vi "Read.ProcessData.vi"(8 "error in (no error)":errorcluster, 10 "timeout ms":i32=100, 11 "Read in":refnum<class "Read.lvclass">) -> (0 "error out":errorcluster, 1 "Timeout?":bool, 2 "Data":dbl[](array[numeric]), 3 "Read out":refnum<class "Read.lvclass">)   [LabVIEW 2015, in "Data Access API.lvlib" / "Read.lvclass"]
uses:
  Read.lvclass
  Read.lvclass/Read.ctl
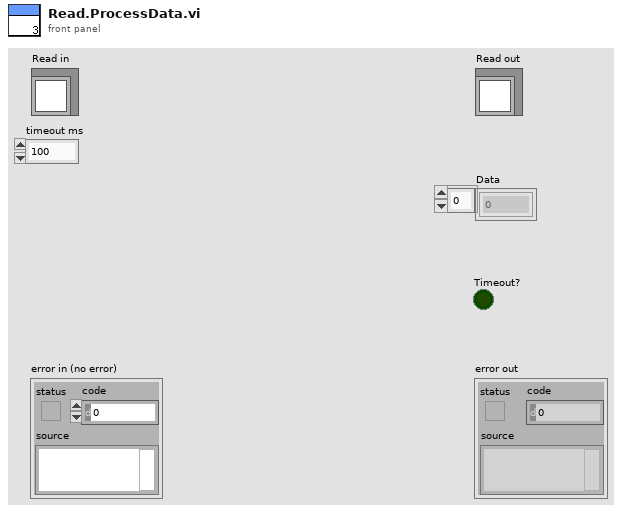
[diagram p1: front panel]
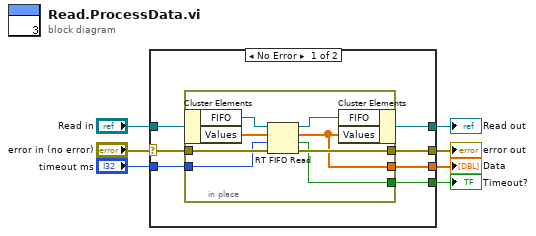
[diagram p0: block diagram]
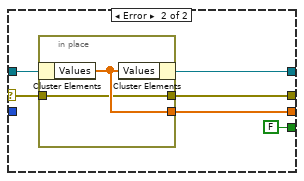
[diagram p2: hidden frame]
diagram:
  n1 = case shown="No Error" "error in (no error)" {
    selector: "error in (no error)" -> [w12 w27]
    tunnel: [w11 w23] -> w6
    tunnel: [w13 w25] -> w4
    tunnel: "Read in" -> [w14 w26]
    tunnel: "timeout ms" -> [w10 _]
    tunnel: [w9 w24] -> w2
    tunnel: [w8 FALSE ("empty?")] -> w1
    frame No Error {
      n2 = in-place {
        in-place-border: w12 -> [w19]
        in-place-border: [w18] -> w11
        in-place-border: w10 -> [w17]
        in-place-border: [w16] -> w9
        in-place-border: [w15] -> w8
        n3 = in-place-cluster #1(w14) -> ("FIFO"=w22:refnum<k33>, "Values"=w20:dbl[])
        n4 = RT FIFO Read(0:w22, 1:w20, 2:w17, 3:w19) -> (8:w21:refnum<k33>, 9:w16:dbl[], 10:w15:bool, 11:w18:errorcluster)  [unwired: 1 out]
        n5 = in-place-cluster #1("FIFO"=w21, "Values"=w16) -> (w13:refnum<class "Read.lvclass">)
      }
    }
    frame Error {
      n6 = in-place {
        in-place-border: w27 -> [w29]
        in-place-border: [w29] -> w23
        in-place-border: [w30] -> w24
        n7 = in-place-cluster #2(w26) -> ("Values"=w30:dbl[])
        n8 = in-place-cluster #2("Values"=w30) -> (w25:refnum<class "Read.lvclass">)
      }
    }
  }
  "error out" <- w6
  "Read out" <- w4
  "Data" <- w2
  "Timeout?" <- w1
